vi "MyMethod1.vi"(0 "reference in":refnum<class "DemoSubSubClass1.lvclass">, 5 "error in (no error)":errorcluster) -> (14 "reference out":refnum<class "DemoSubSubClass1.lvclass">, 19 "error out":errorcluster)   [LabVIEW 2020, in "DemoSubSubClass1.lvclass"]
uses:
  DemoSubSubClass1.lvclass
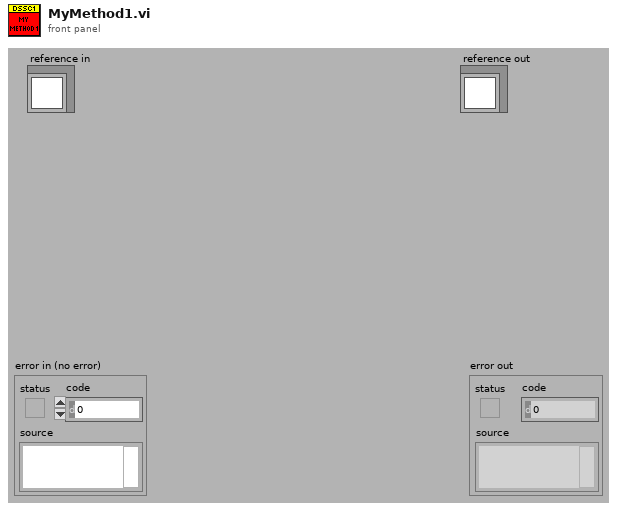
[diagram p1: front panel]
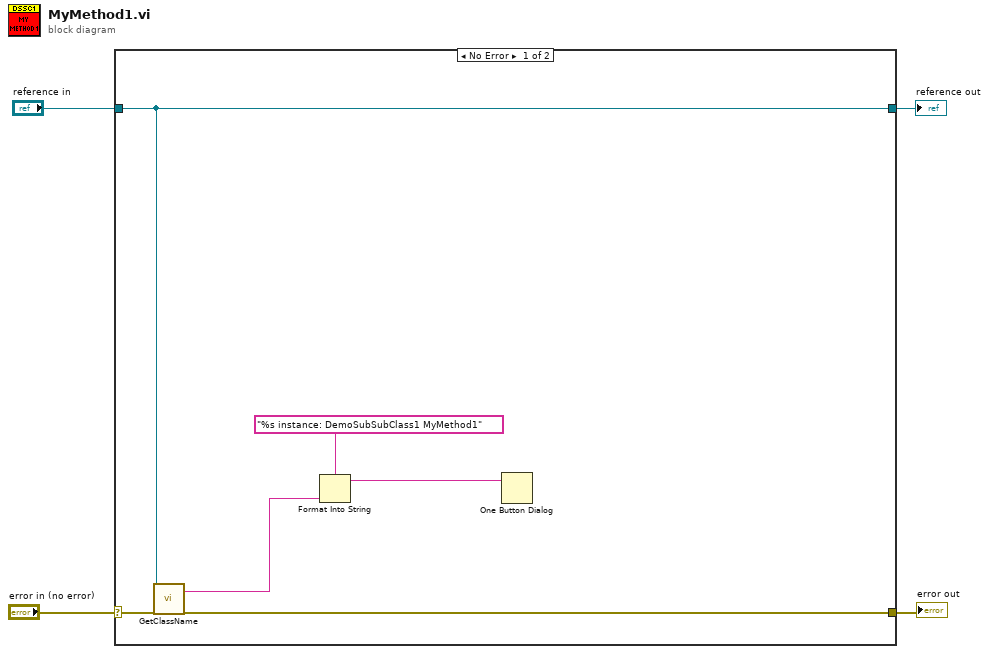
[diagram p0: block diagram]
diagram:
  n1 = case shown="No Error" "error in (no error)" {
    selector: "error in (no error)" -> [w10 w12]
    tunnel: [w9 w12] -> w3
    tunnel: [w8 w11] -> w1
    tunnel: "reference in" -> [w8 w11]
    frame No Error {
      n2 = call-dynamic "GetClassName.vi"("reference in"=w8, "error in (no error)"=w10) -> ("class name"=w6:string, "error out"=w9:errorcluster)  [unwired: 13 in, 3 out]
      n3 = Format Into String(format string="%s instance: DemoSubSubClass1 MyMethod1" ("message"), w6) -> (resulting string=w5:string)  [unwired: 2 in, 1 out]
      n4 = One Button Dialog(message=w5) -> ()  [unwired: 2 out]
    }
    frame Error {
    }
  }
  "error out" <- w3
  "reference out" <- w1
